vi "Initialize AO Task.vi"(8 "error in (no error)":errorcluster, 11 "BNT_DAQmx-MCSV in":refnum<class "BNT_DAQmx-MCSV.lvclass">) -> (0 "error out":errorcluster, 3 "AO DAQmx Task":refnum<k21>)   [LabVIEW 2017, in "BNT_DAQmx.lvlib" / "BNT_DAQmx-MCSV.lvclass"]
doc: "Initialize DAQmx Analog Input task.\n\n<b>Default Implementation:</b> Analog Input Voltage\n\nThis dynamic dispatch VI can be overritten by derived classes to implement other analog input tasks."
uses:
  BNT_DAQmx-MCSV.lvclass
  C:/User/Brand/LVP/Acc/VacuumHeating/Packages/CSPP_Core/Actors/CSPP_BaseActor/CSPP_BaseActor.lvclass
  CSPP_Core/Actors/CSPP_BaseActor/CSPP_BaseActor.lvclass/CSPP_BaseActor.ctl
  BNT_DAQmx-MCSV.lvclass/BNT_DAQmx-MCSV.ctl
  <vilib>/DAQmx/create/channels.llb/DAQmx Create Channel (AO-Voltage-Basic).vi
  CSPP_Core/Actors/CSPP_BaseActor/CSPP_BaseActor.lvclass
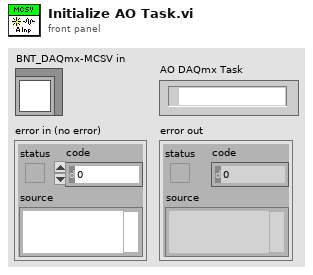
[diagram p1: front panel]
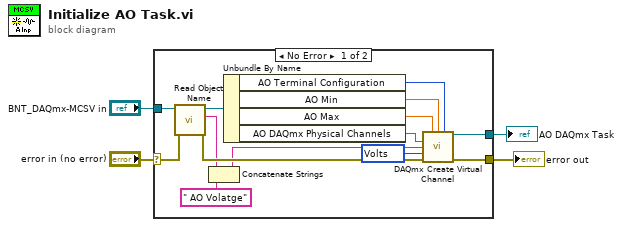
[diagram p0: block diagram]
diagram:
  n1 = case shown="No Error" "error in (no error)" {
    selector: "error in (no error)" -> [w9 w19]
    tunnel: [w16 w19] -> w3
    tunnel: "BNT_DAQmx-MCSV in" -> [w11 _]
    tunnel: [w14 _] -> w1
    frame No Error {
      w15 = 10348 items=["Volts"=10348, "From Custom Scale"=10065] ("units")
      n2 = call "Read Object Name.vi"("error in (no error)"=w9, "CSPP_BaseActor in"=w11) -> ("error out"=w8:errorcluster, "Object Name"=w6:string, "CSPP_BaseActor out"=w10:refnum<class "BNT_DAQmx-MCSV.lvclass">)  [unwired: 7 in]
      n3 = Concatenate Strings(w6, " AO Volatge" ("string")) -> (w5:string)
      n4 = Unbundle By Name(w10) -> ("AO Terminal Configuration"=w18:i32, "AO Min"=w13:dbl, "AO Max"=w12:dbl, "AO DAQmx Physical Channels"=w17:tag)
      n5 = call-poly <vilib>:"DAQmx Create Virtual Channel.vi"("maximum value"=w12, "minimum value"=w13, "output terminal configuration"=w18, "physical channels"=w17, "name to assign"=w5, "units"=w15, "error in"=w8) -> ("task out"=w14:refnum<k21>, "error out"=w16:errorcluster)  [unwired: 7 in]
    }
    frame Error {
    }
  }
  "error out" <- w3
  "AO DAQmx Task" <- w1
